vi "DisableControls.vi"(7 "Enable (T)":bool, 8 "error in (no error)":errorcluster, 10 "Device Properties In":T1={"Configuration Mode"=enum."Constant Power (AC)", "Phases"=[{"Handle"="", "Name"="", "Phase Select"=1, "Instrument Options"="", "id query (T)"=TRUE, "reset device (T)"=TRUE, "Load Short Circuited"=FALSE, "Line Synchronization"=FALSE, "Load Current (A/Arms)"=1.0, "Load Voltage (V/Vrms)"=0.0, "Load Power (W)"=0.0, "Load Resistance (Ohms)"=0.0, "Load Current Peak Limit (A)"=0.0, "Load Current Limit (A/Arms)"=0.0, "Load Power Limit (W)"=0.0, "Synch Frequency (Hz)"=0.0, "Priority"=enum."CF Only", "Crest Factor"=0.0, "Power Factor"=0.0, "Slew Rate"={"Rise Slew Rate (A/ms)"=0, "Fall Slew Rate (A/ms)"=0}, "LC/RLC Mode"={"Capacitance (uF)"=0, "Inductance (uH)"=0, "Series Resistance (Ohm)"=0.0, "Parallel Resistance (Ohm)"=0.0}, "Timing"={"TimingOn"=enum."", "Hours"=0, "Minutes"=0, "Seconds"=0.0, "CutoffVoltage"=0.0}, "Connected"=FALSE}], "MeasName"=""} {"Phases"."Phase Select" items=["Phase ALL", "Phase A", "Phase B", "Phase C"]; "Phases"."Slew Rate"."Fall Slew Rate (A/ms)" min=4 max=600 step=1; "Phases"."Slew Rate"."Rise Slew Rate (A/ms)" min=4 max=600 step=1}, 11 "Cluster":refnum<vi>) -> (0 "Error Out":errorcluster, 2 "Device Properties Out":T1={"Configuration Mode"=enum."Constant Power (AC)", "Phases"=[{"Handle"="", "Name"="", "Phase Select"=1, "Instrument Options"="", "id query (T)"=TRUE, "reset device (T)"=TRUE, "Load Short Circuited"=FALSE, "Line Synchronization"=FALSE, "Load Current (A/Arms)"=1.0, "Load Voltage (V/Vrms)"=0.0, "Load Power (W)"=0.0, "Load Resistance (Ohms)"=0.0, "Load Current Peak Limit (A)"=0.0, "Load Current Limit (A/Arms)"=0.0, "Load Power Limit (W)"=0.0, "Synch Frequency (Hz)"=0.0, "Priority"=enum."CF Only", "Crest Factor"=0.0, "Power Factor"=0.0, "Slew Rate"={"Rise Slew Rate (A/ms)"=0, "Fall Slew Rate (A/ms)"=0}, "LC/RLC Mode"={"Capacitance (uF)"=0, "Inductance (uH)"=0, "Series Resistance (Ohm)"=0.0, "Parallel Resistance (Ohm)"=0.0}, "Timing"={"TimingOn"=enum."", "Hours"=0, "Minutes"=0, "Seconds"=0.0, "CutoffVoltage"=0.0}, "Connected"=FALSE}], "MeasName"=""} {"Phases"."Phase Select" items=["Phase ALL", "Phase A", "Phase B", "Phase C"]; "Phases"."Slew Rate"."Fall Slew Rate (A/ms)" min=4 max=600 step=1; "Phases"."Slew Rate"."Rise Slew Rate (A/ms)" min=4 max=600 step=1})   [LabVIEW 2018, in "AcPwrPlugins.lvlib" / "ChromaAcLoad.lvclass"]
doc: "This VI disables the controls in the phases cluster based on the Configuration Mode control. This will enable the user to only change the values of the controls that are allowed by that mode."
uses:
  ChromaAcLoad.lvclass
  TypeDefs/Device(s)Settings.ctl
  TypeDefs/ConfigMode.ctl
panel:
  # "1"
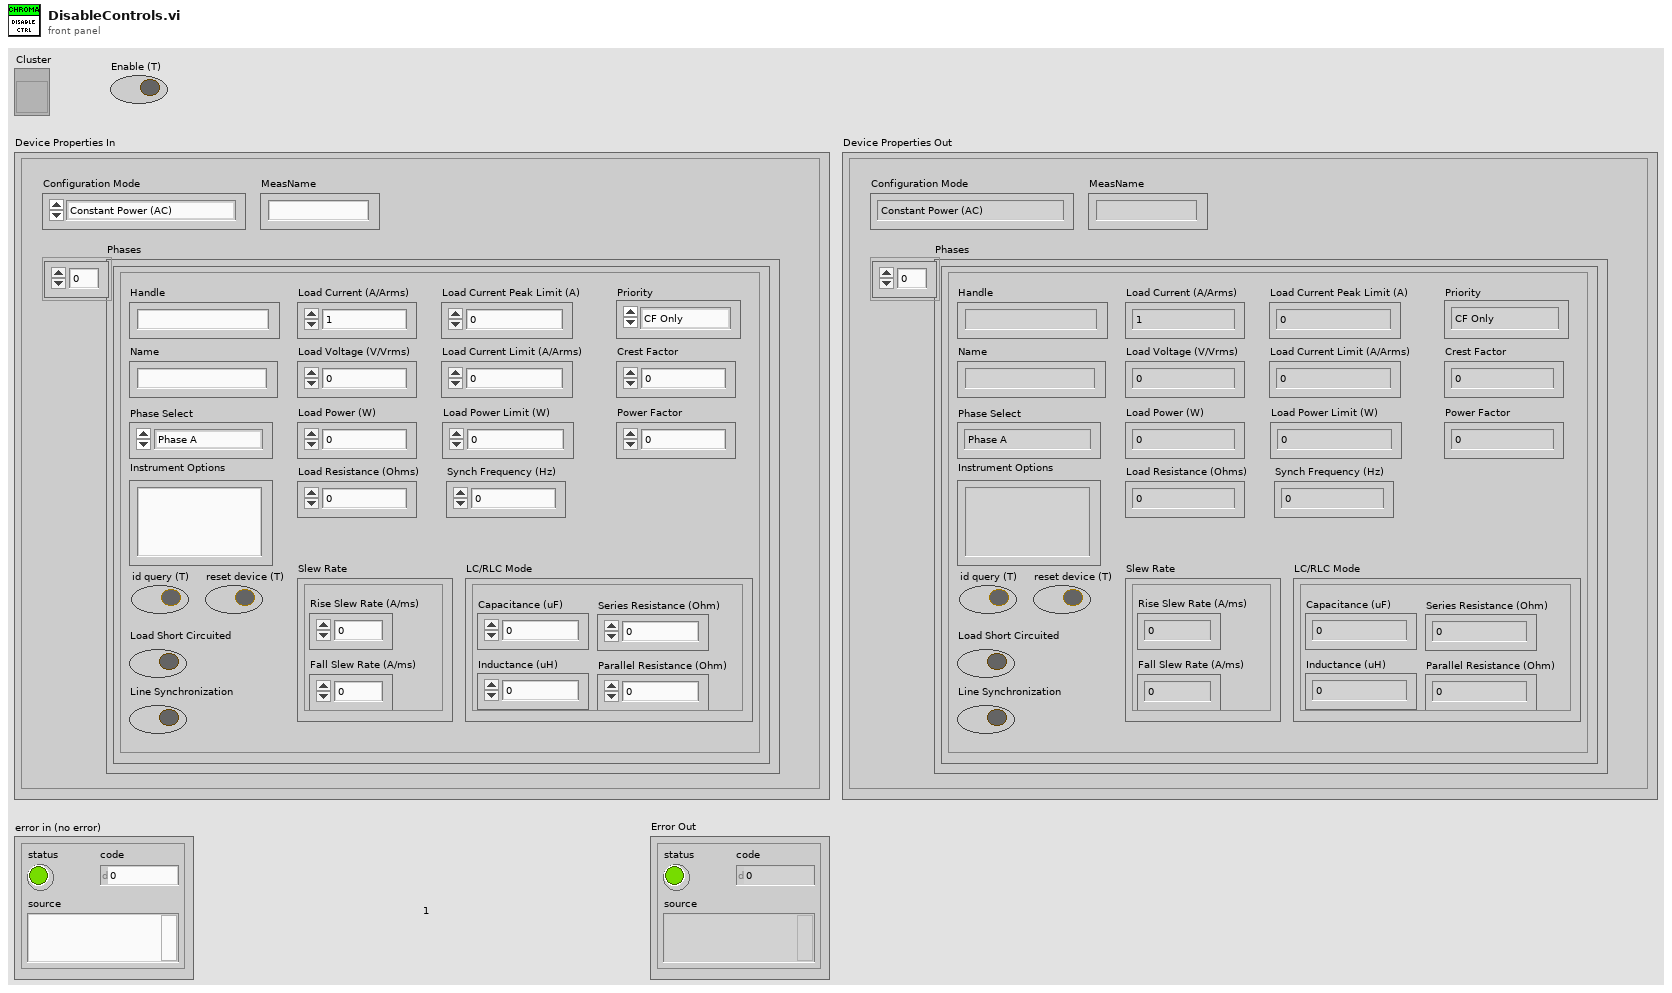
[diagram p1: front panel]
types:
  T1 = typedef "AcPwrPlugins.lvlib/ChromaAcLoad.lvclass/Device(s)Settings.ctl" = cluster{"Configuration Mode":T2, "Phases":cluster{"Handle":string, "Name":string, "Phase Select":i32, "Instrument Options":string, "id query (T)":bool, "reset device (T)":bool, "Load Short Circuited":bool, "Line Synchronization":bool, "Load Current (A/Arms)":dbl, "Load Voltage (V/Vrms)":dbl, "Load Power (W)":dbl, "Load Resistance (Ohms)":dbl, "Load Current Peak Limit (A)":dbl, "Load Current Limit (A/Arms)":dbl, "Load Power Limit (W)":dbl, "Synch Frequency (Hz)":dbl, "Priority":enum16{"CF Only", "PF Only", "Both (CF)", "Both (PF)"}, "Crest Factor":dbl, "Power Factor":dbl, "Slew Rate":cluster{"Rise Slew Rate (A/ms)":i32, "Fall Slew Rate (A/ms)":i32}, "LC/RLC Mode":cluster{"Capacitance (uF)":i32, "Inductance (uH)":i32, "Series Resistance (Ohm)":dbl, "Parallel Resistance (Ohm)":dbl}, "Timing":cluster{"TimingOn":enum16{""}, "Hours":u32, "Minutes":u32, "Seconds":dbl, "CutoffVoltage":dbl}, "Connected":bool}[], "MeasName":string}
  T2 = typedef "ConfigMode.ctl" = enum16{"Constant Voltage (DC)", "Constant Power (DC)", "Constant Power (AC)", "Constant Current (DC)", "Constant Current (AC)", "Constant Resistance (DC)", "Constant Resistance (AC)", "Rectified Mode (DC)", "Inrush (AC)", "RLC CP (AC)", "RLC (AC)"}
  T3 = enum8{"Enabled", "Disabled", "Disabled and Grayed Out"}
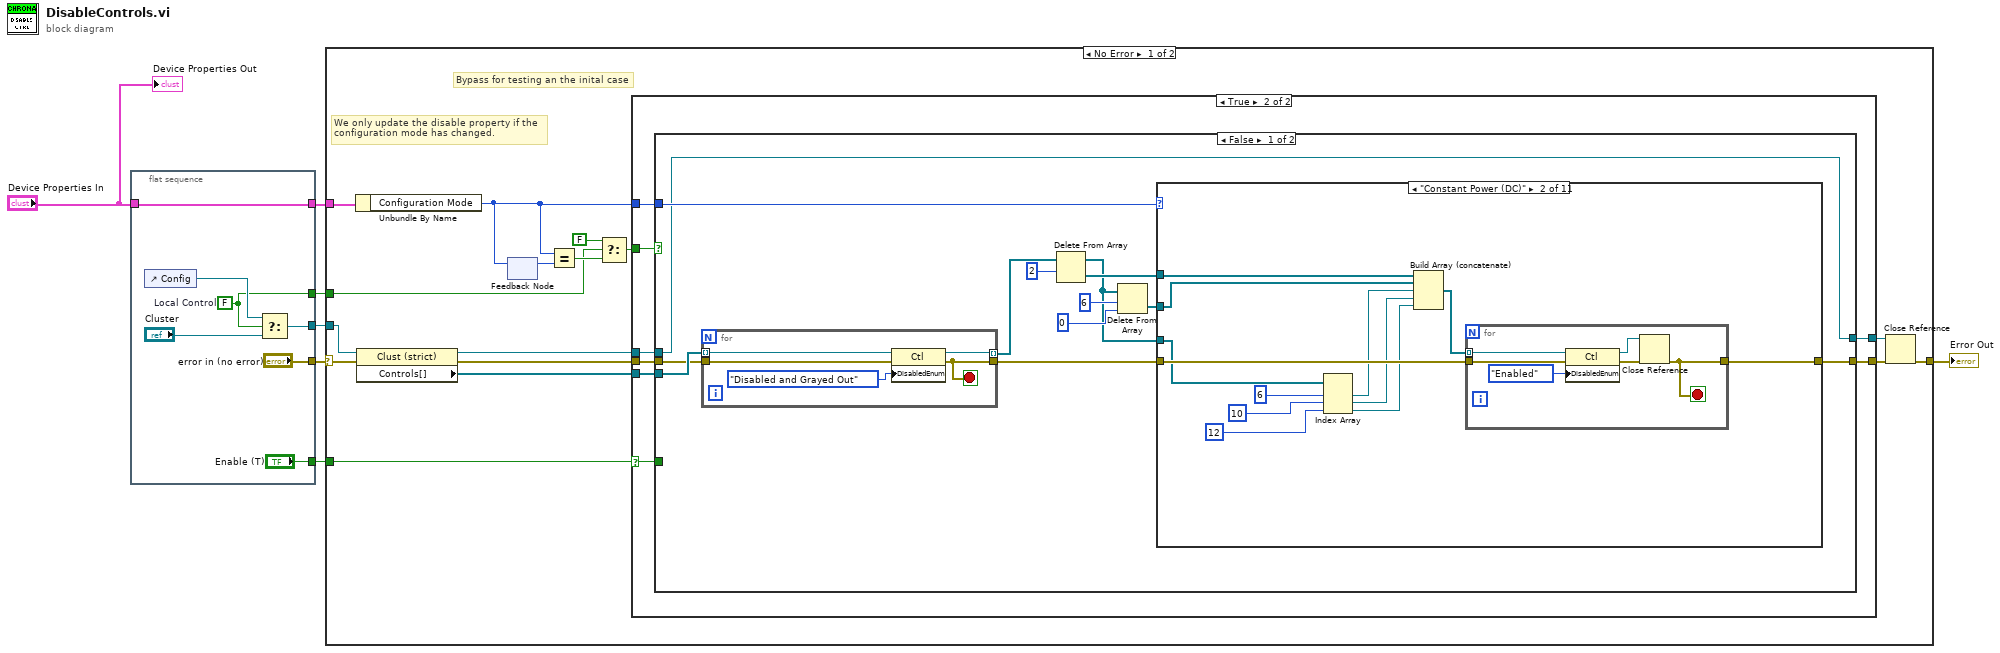
[diagram p0: block diagram]
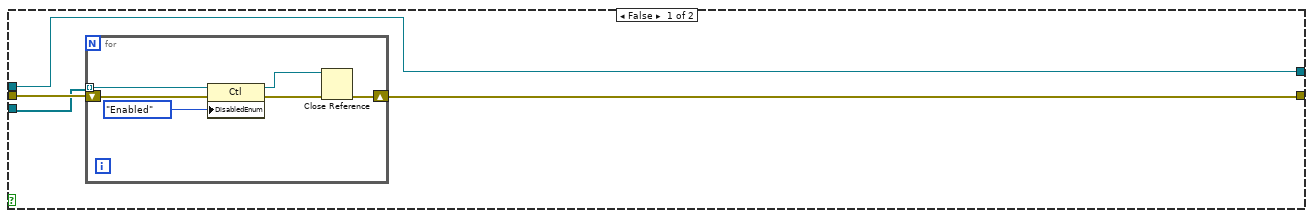
[diagram p2: hidden frame]
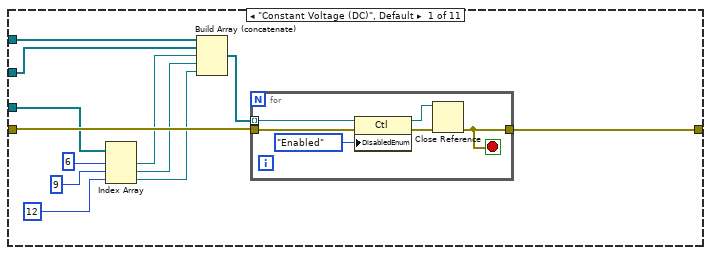
[diagram p3: hidden frame]
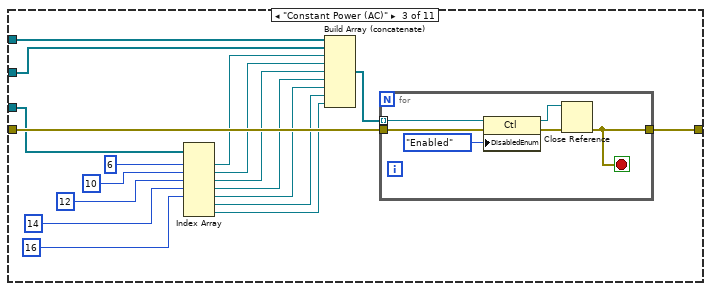
[diagram p4: hidden frame]
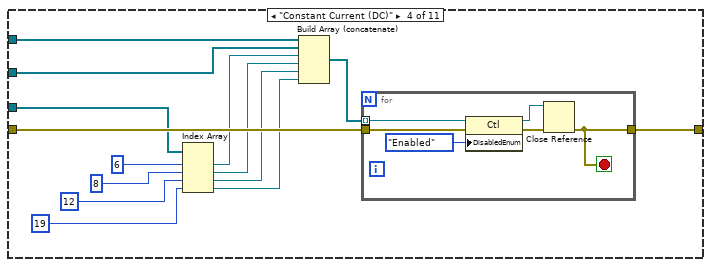
[diagram p5: hidden frame]
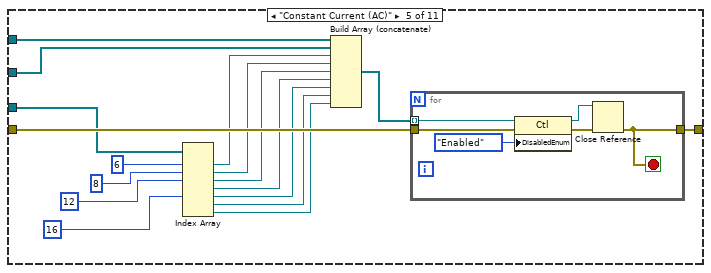
[diagram p6: hidden frame]
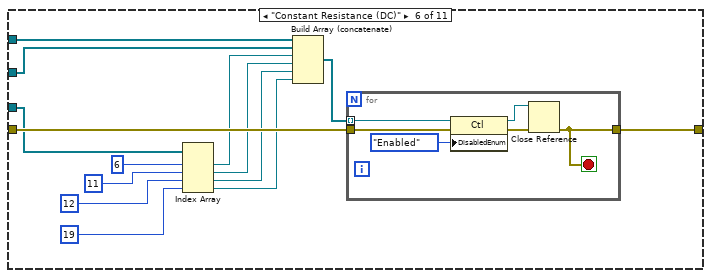
[diagram p7: hidden frame]
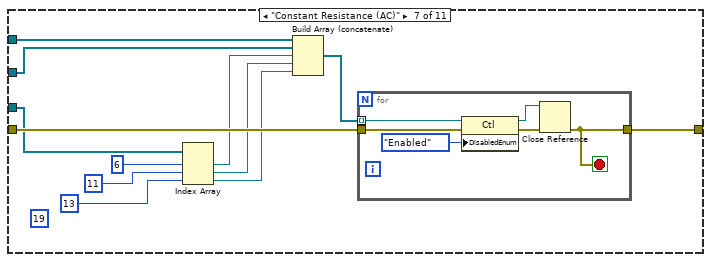
[diagram p8: hidden frame]
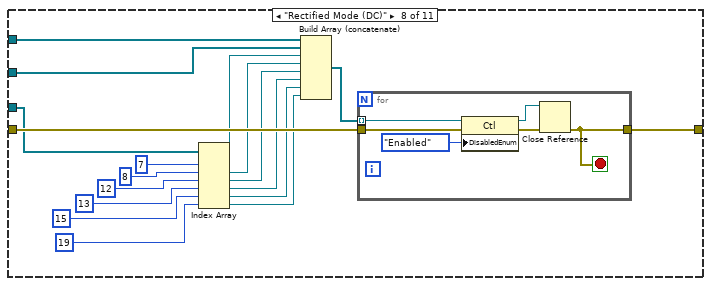
[diagram p9: hidden frame]
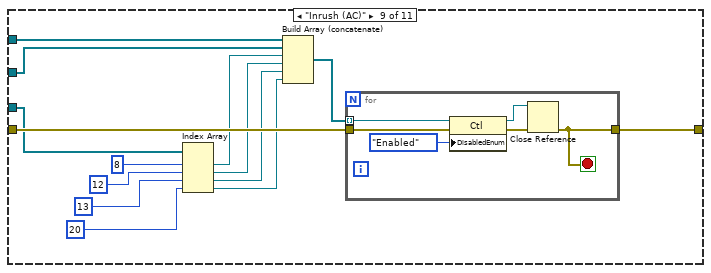
[diagram p10: hidden frame]
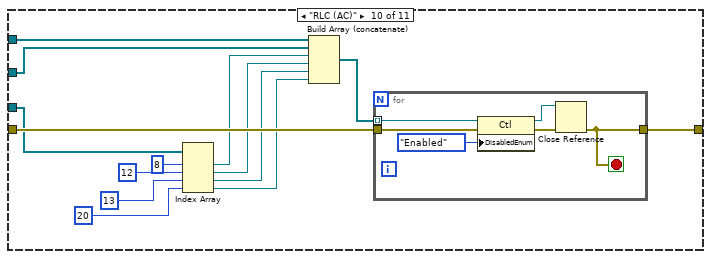
[diagram p11: hidden frame]
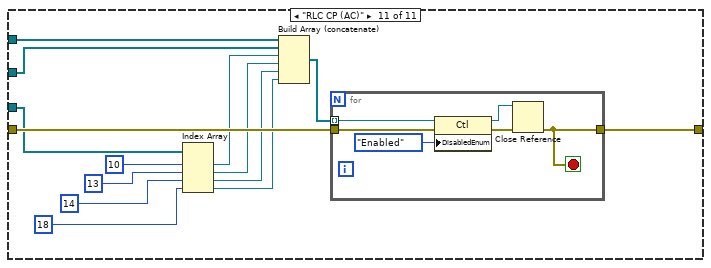
[diagram p12: hidden frame]
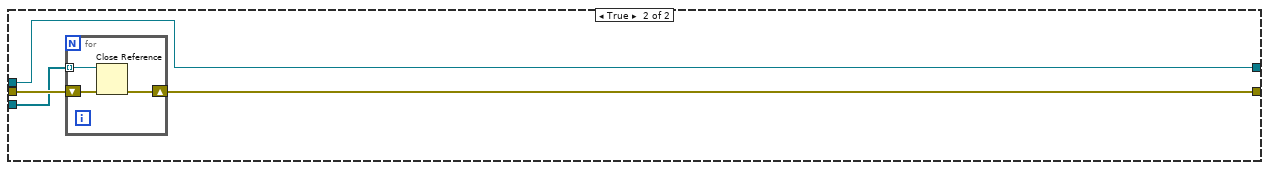
[diagram p13: hidden frame]
diagram:
  n1 = flat-sequence {
    tunnel: ["error in (no error)"] -> w6
    tunnel: [w13] -> w5
    tunnel: [w9] -> w4
    tunnel: ["Enable (T)"] -> w3
    tunnel: "Device Properties In" -> [w10]
    tunnel: [w10] -> w1
    frame #0 {
      w9 = FALSE  # Local Control
      n2 = control-ref of="Config"() -> (w11:refnum<vi>)
      n3 = Select(t=w11, s=w9, f="Cluster") -> (s? t:f=w13:refnum<vi>)
    }
  }
  n4 = case shown="No Error" w6 {
    selector: w6 -> [w24 w299]
    tunnel: [w23 w299] -> w7
    tunnel: w5 -> [w26 _]
    tunnel: w4 -> [w16 _]
    tunnel: w3 -> [w18 _]
    tunnel: w1 -> [w17 _]
    frame No Error {
      # "Bypass for testing an the inital case"
      # "We only update the disable property if the\nconfiguration mode has changed."
      n5 = Unbundle By Name(w17) -> ("Configuration Mode"=w25:T2)
      n6 = property class="Clust (strict)"(reference=w26, error in=w24) -> (reference out=w28:refnum<vi>, error out=w29:errorcluster, "Controls[]"=w27:refnum<vi>[])
      n7 = feedback #1() -> (w15:T2)  [unwired: 1 in]
      n8 = feedback-in #1(w25) -> ()
      n9 = Equal?(x=w25, y=w15) -> (x = y?=w21:bool)
      n10 = Select(t=FALSE, s=w16, f=w21) -> (s? t:f=w20:bool)
      n11 = case shown="True" w18 {
        selector: w18 -> [_ w47]
        tunnel: [w32 w48] -> w30
        tunnel: w29 -> [w34 w46]
        tunnel: w28 -> [w31 w45]
        tunnel: w27 -> [w33 w44]
        tunnel: w25 -> [_ w43]
        tunnel: w20 -> [_ w42]
        tunnel: [w31 w41] -> w22
        frame False {
          n12 = for {
            shift-right: [w36] -> w32
            shift-left: w34 -> [w39]
            tunnel: w33 -> [w38] mode=indexing
            n13 = property on="Property Node" class="Ctl"(reference=w38, error in=w39, "DisabledEnum"=T3."Enabled" ("Disabled")) -> (reference out=w35:refnum<vi>, error out=w37:errorcluster)
            n14 = Close Reference(reference=w35, error in (no error)=w37) -> (error out=w36:errorcluster)
          }
        }
        frame True {
          n15 = case shown="False" w42 {
            tunnel: [w61 w293] -> w48
            tunnel: w46 -> [w49 w295]
            tunnel: w45 -> [w52 w292]
            tunnel: w44 -> [w51 w294]
            tunnel: w43 -> [w59 _]
            tunnel: [w52 w292] -> w41
            tunnel: w47 -> [_ _]
            frame False {
              n16 = for {
                tunnel: [w65] -> w50 mode=indexing
                tunnel: w51 -> [w64] mode=indexing
                tunnel: w49 -> [w63]
                tunnel: [w62] -> w60
                stop <- w62 stop-if-true
                n17 = property class="Ctl"(reference=w64, error in=w63, "DisabledEnum"=T3."Disabled and Grayed Out" ("Disabled")) -> (reference out=w65:refnum<vi>, error out=w62:errorcluster)
              }
              n18 = Delete From Array(array=w50, length=2) -> (deleted portion=w55:refnum<vi>[], array with subset deleted=w53:refnum<vi>[])  [unwired: 1 in]
              n19 = Delete From Array(array=w53, length=6, index=0) -> (deleted portion=w54:refnum<vi>[])  [unwired: 1 out]
              n20 = case shown="\"Constant Power (DC)\"" w59 {
                tunnel: [w77 w95 w119 w139 w162 w182 w200 w224 w244 w264 w284] -> w61
                tunnel: w60 -> [w78 w96 w120 w140 w163 w183 w201 w225 w245 w265 w285]
                tunnel: w55 -> [w69 w87 w107 w129 w150 w172 w192 w214 w239 w257 w276]
                tunnel: w54 -> [w68 w86 w106 w128 w149 w171 w191 w213 w238 w256 w275]
                tunnel: w53 -> [w67 w85 w105 w127 w148 w170 w190 w212 w237 w255 w274]
                frame "Constant Voltage (DC)", Default {
                  n21 = Index Array(array=w67, index #1=6 ("index"), index #2=9 ("index"), index #3=12 ("index")) -> (element #1=w74:refnum<vi>, element #2=w73:refnum<vi>, element #3=w71:refnum<vi>)
                  n22 = Build Array (concatenate)(w69, w68, w74, w73, w71) -> (w76:refnum<vi>[])
                  n23 = for {
                    tunnel: w78 -> [w84]
                    tunnel: [w79] -> w77
                    tunnel: w76 -> [w82] mode=indexing
                    stop <- w79 stop-if-true
                    n24 = property class="Ctl"(reference=w82, error in=w84, "DisabledEnum"=T3."Enabled" ("Disabled")) -> (reference out=w80:refnum<vi>, error out=w81:errorcluster)
                    n25 = Close Reference(reference=w80, error in (no error)=w81) -> (error out=w79:errorcluster)
                  }
                }
                frame "Constant Power (DC)" {
                  n26 = Index Array(array=w85, index #1=6 ("index"), index #2=10 ("index"), index #3=12 ("index")) -> (element #1=w92:refnum<vi>, element #2=w91:refnum<vi>, element #3=w88:refnum<vi>)
                  n27 = Build Array (concatenate)(w87, w86, w92, w91, w88) -> (w94:refnum<vi>[])
                  n28 = for {
                    tunnel: w96 -> [w102]
                    tunnel: [w97] -> w95
                    tunnel: w94 -> [w100] mode=indexing
                    stop <- w97 stop-if-true
                    n29 = property class="Ctl"(reference=w100, error in=w102, "DisabledEnum"=T3."Enabled" ("Disabled")) -> (reference out=w98:refnum<vi>, error out=w99:errorcluster)
                    n30 = Close Reference(reference=w98, error in (no error)=w99) -> (error out=w97:errorcluster)
                  }
                }
                frame "Constant Power (AC)" {
                  n31 = Index Array(array=w105, index #1=6 ("index"), index #2=10 ("index"), index #3=12 ("index"), index #4=14 ("index"), index #5=16 ("index")) -> (element #1=w116:refnum<vi>, element #2=w115:refnum<vi>, element #3=w113:refnum<vi>, element #4=w110:refnum<vi>, element #5=w109:refnum<vi>, element #6=w108:refnum<vi>, element #7=w103:refnum<vi>)  [unwired: 2 in]
                  n32 = Build Array (concatenate)(w107, w106, w116, w115, w113, w110, w109, w108, w103) -> (w118:refnum<vi>[])
                  n33 = for {
                    tunnel: w120 -> [w126]
                    tunnel: [w121] -> w119
                    tunnel: w118 -> [w124] mode=indexing
                    stop <- w121 stop-if-true
                    n34 = property class="Ctl"(reference=w124, error in=w126, "DisabledEnum"=T3."Enabled" ("Disabled")) -> (reference out=w122:refnum<vi>, error out=w123:errorcluster)
                    n35 = Close Reference(reference=w122, error in (no error)=w123) -> (error out=w121:errorcluster)
                  }
                }
                frame "Constant Current (DC)" {
                  n36 = Index Array(array=w127, index #1=6 ("index"), index #2=8 ("index"), index #3=12 ("index"), index #4=19 ("index")) -> (element #1=w136:refnum<vi>, element #2=w135:refnum<vi>, element #3=w133:refnum<vi>, element #4=w130:refnum<vi>)
                  n37 = Build Array (concatenate)(w129, w128, w136, w135, w133, w130) -> (w138:refnum<vi>[])
                  n38 = for {
                    tunnel: w140 -> [w146]
                    tunnel: [w141] -> w139
                    tunnel: w138 -> [w144] mode=indexing
                    stop <- w141 stop-if-true
                    n39 = property class="Ctl"(reference=w144, error in=w146, "DisabledEnum"=T3."Enabled" ("Disabled")) -> (reference out=w142:refnum<vi>, error out=w143:errorcluster)
                    n40 = Close Reference(reference=w142, error in (no error)=w143) -> (error out=w141:errorcluster)
                  }
                }
                frame "Constant Current (AC)" {
                  n41 = Index Array(array=w148, index #1=6 ("index"), index #2=8 ("index"), index #3=12 ("index"), index #5=16 ("index")) -> (element #1=w159:refnum<vi>, element #2=w158:refnum<vi>, element #3=w156:refnum<vi>, element #4=w154:refnum<vi>, element #5=w153:refnum<vi>, element #6=w152:refnum<vi>, element #7=w151:refnum<vi>)  [unwired: 3 in]
                  n42 = Build Array (concatenate)(w150, w149, w159, w158, w156, w154, w153, w152, w151) -> (w161:refnum<vi>[])
                  n43 = for {
                    tunnel: w163 -> [w169]
                    tunnel: [w164] -> w162
                    tunnel: w161 -> [w167] mode=indexing
                    stop <- w164 stop-if-true
                    n44 = property class="Ctl"(reference=w167, error in=w169, "DisabledEnum"=T3."Enabled" ("Disabled")) -> (reference out=w165:refnum<vi>, error out=w166:errorcluster)
                    n45 = Close Reference(reference=w165, error in (no error)=w166) -> (error out=w164:errorcluster)
                  }
                }
                frame "Constant Resistance (DC)" {
                  n46 = Index Array(array=w170, index #1=6 ("index"), index #2=11 ("index"), index #3=12 ("index"), index #4=19 ("index")) -> (element #1=w179:refnum<vi>, element #2=w178:refnum<vi>, element #3=w175:refnum<vi>, element #4=w173:refnum<vi>)
                  n47 = Build Array (concatenate)(w172, w171, w179, w178, w175, w173) -> (w181:refnum<vi>[])
                  n48 = for {
                    tunnel: w183 -> [w189]
                    tunnel: [w184] -> w182
                    tunnel: w181 -> [w187] mode=indexing
                    stop <- w184 stop-if-true
                    n49 = property class="Ctl"(reference=w187, error in=w189, "DisabledEnum"=T3."Enabled" ("Disabled")) -> (reference out=w185:refnum<vi>, error out=w186:errorcluster)
                    n50 = Close Reference(reference=w185, error in (no error)=w186) -> (error out=w184:errorcluster)
                  }
                }
                frame "Constant Resistance (AC)" {
                  (unwired) 19 ("index")
                  n51 = Index Array(array=w190, index #1=6 ("index"), index #2=11 ("index"), index #3=13 ("index")) -> (element #1=w197:refnum<vi>, element #2=w196:refnum<vi>, element #3=w193:refnum<vi>)
                  n52 = Build Array (concatenate)(w192, w191, w197, w196, w193) -> (w199:refnum<vi>[])
                  n53 = for {
                    tunnel: w201 -> [w207]
                    tunnel: [w202] -> w200
                    tunnel: w199 -> [w205] mode=indexing
                    stop <- w202 stop-if-true
                    n54 = property class="Ctl"(reference=w205, error in=w207, "DisabledEnum"=T3."Enabled" ("Disabled")) -> (reference out=w203:refnum<vi>, error out=w204:errorcluster)
                    n55 = Close Reference(reference=w203, error in (no error)=w204) -> (error out=w202:errorcluster)
                  }
                }
                frame "Rectified Mode (DC)" {
                  n56 = Index Array(array=w212, index #1=7 ("index"), index #2=8 ("index"), index #3=12 ("index"), index #4=13 ("index"), index #5=15 ("index"), index #6=19 ("index")) -> (element #1=w221:refnum<vi>, element #2=w220:refnum<vi>, element #3=w217:refnum<vi>, element #4=w215:refnum<vi>, element #5=w211:refnum<vi>, element #6=w208:refnum<vi>)
                  n57 = Build Array (concatenate)(w214, w213, w221, w220, w217, w215, w211, w208) -> (w223:refnum<vi>[])
                  n58 = for {
                    tunnel: w225 -> [w231]
                    tunnel: [w226] -> w224
                    tunnel: w223 -> [w229] mode=indexing
                    stop <- w226 stop-if-true
                    n59 = property class="Ctl"(reference=w229, error in=w231, "DisabledEnum"=T3."Enabled" ("Disabled")) -> (reference out=w227:refnum<vi>, error out=w228:errorcluster)
                    n60 = Close Reference(reference=w227, error in (no error)=w228) -> (error out=w226:errorcluster)
                  }
                }
                frame "Inrush (AC)" {
                  n61 = Index Array(array=w237, index #1=8 ("index"), index #2=12 ("index"), index #3=13 ("index"), index #4=20 ("index")) -> (element #1=w242:refnum<vi>, element #2=w241:refnum<vi>, element #3=w240:refnum<vi>, element #4=w232:refnum<vi>)
                  n62 = Build Array (concatenate)(w239, w238, w242, w241, w240, w232) -> (w243:refnum<vi>[])
                  n63 = for {
                    tunnel: w245 -> [w251]
                    tunnel: [w246] -> w244
                    tunnel: w243 -> [w249] mode=indexing
                    stop <- w246 stop-if-true
                    n64 = property class="Ctl"(reference=w249, error in=w251, "DisabledEnum"=T3."Enabled" ("Disabled")) -> (reference out=w247:refnum<vi>, error out=w248:errorcluster)
                    n65 = Close Reference(reference=w247, error in (no error)=w248) -> (error out=w246:errorcluster)
                  }
                }
                frame "RLC (AC)" {
                  n66 = Index Array(array=w255, index #1=8 ("index"), index #2=12 ("index"), index #3=13 ("index"), index #4=20 ("index")) -> (element #1=w261:refnum<vi>, element #2=w260:refnum<vi>, element #3=w259:refnum<vi>, element #4=w258:refnum<vi>)
                  n67 = Build Array (concatenate)(w257, w256, w261, w260, w259, w258) -> (w263:refnum<vi>[])
                  n68 = for {
                    tunnel: w265 -> [w271]
                    tunnel: [w266] -> w264
                    tunnel: w263 -> [w269] mode=indexing
                    stop <- w266 stop-if-true
                    n69 = property class="Ctl"(reference=w269, error in=w271, "DisabledEnum"=T3."Enabled" ("Disabled")) -> (reference out=w267:refnum<vi>, error out=w268:errorcluster)
                    n70 = Close Reference(reference=w267, error in (no error)=w268) -> (error out=w266:errorcluster)
                  }
                }
                frame "RLC CP (AC)" {
                  n71 = Index Array(array=w274, index #1=10 ("index"), index #2=13 ("index"), index #3=14 ("index"), index #4=18 ("index")) -> (element #1=w281:refnum<vi>, element #2=w280:refnum<vi>, element #3=w277:refnum<vi>, element #4=w272:refnum<vi>)
                  n72 = Build Array (concatenate)(w276, w275, w281, w280, w277, w272) -> (w283:refnum<vi>[])
                  n73 = for {
                    tunnel: w285 -> [w291]
                    tunnel: [w286] -> w284
                    tunnel: w283 -> [w289] mode=indexing
                    stop <- w286 stop-if-true
                    n74 = property class="Ctl"(reference=w289, error in=w291, "DisabledEnum"=T3."Enabled" ("Disabled")) -> (reference out=w287:refnum<vi>, error out=w288:errorcluster)
                    n75 = Close Reference(reference=w287, error in (no error)=w288) -> (error out=w286:errorcluster)
                  }
                }
              }
            }
            frame True {
              n76 = for {
                shift-right: [w296] -> w293
                shift-left: w295 -> [w298]
                tunnel: w294 -> [w297] mode=indexing
                n77 = Close Reference(reference=w297, error in (no error)=w298) -> (error out=w296:errorcluster)
              }
            }
          }
        }
      }
      n78 = Close Reference(reference=w22, error in (no error)=w30) -> (error out=w23:errorcluster)
    }
    frame Error {
    }
  }
  "Error Out" <- w7
  "Device Properties Out" <- "Device Properties In"
